vi "IniRW.vi"(6 "WriteIfNotExists":bool=TRUE, 7 "Operation":enum16{"None", "Read", "Write"}(ring)=enum."Read", 8 "InputValue":string, 9 "Key":string, 10 "Section":string, 11 "IniFilePath":path) -> (0 "IsValidFile":bool, 2 "OutputValue":string, 3 "IniFilePath out":path)   [LabVIEW 2024]
uses:
  <vilib>/Utility/config.llb/Read Key (String).vi
  <vilib>/Utility/config.llb/Write Key (String).vi
  <vilib>/Utility/config.llb/NI_LVConfig.lvlib
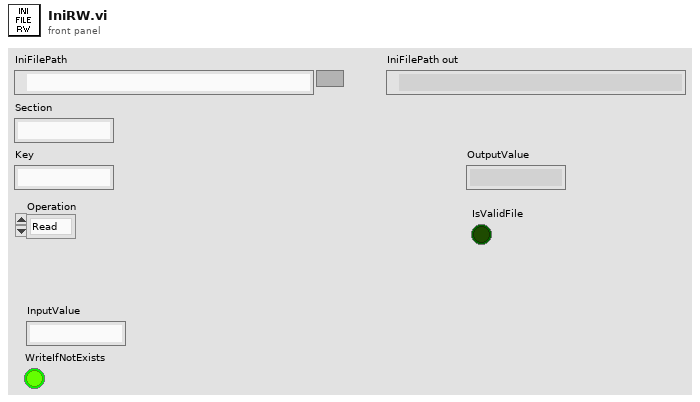
[diagram p1: front panel]
types:
  T1 = typedef "NI_LVConfig.lvlib/Config Data RefNum.ctl" = refnum<k1>
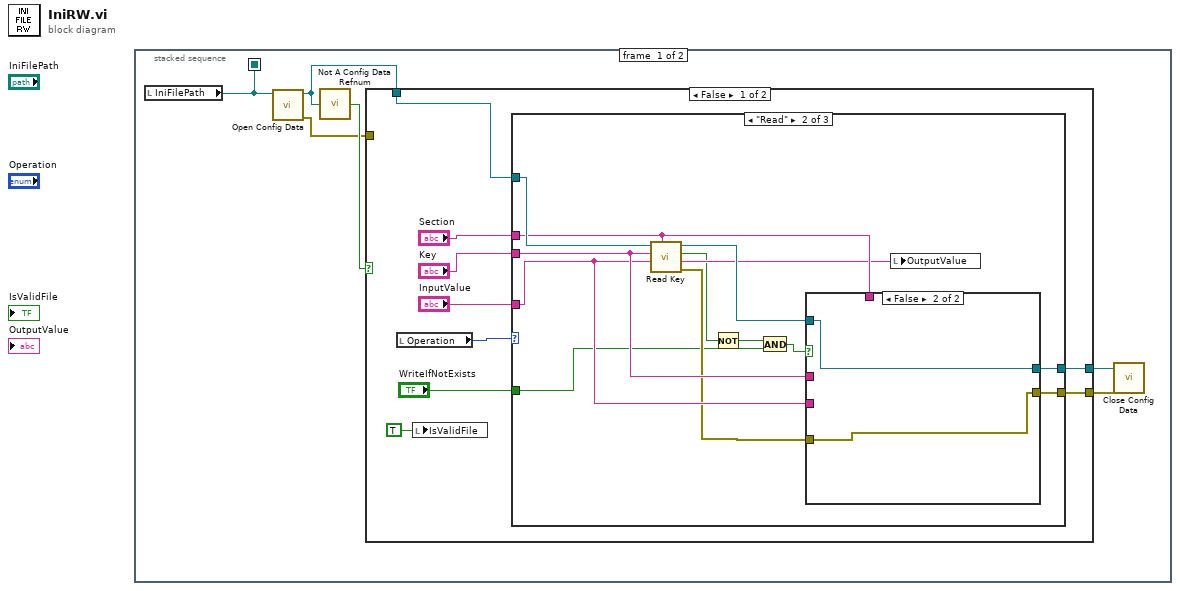
[diagram p0: block diagram]
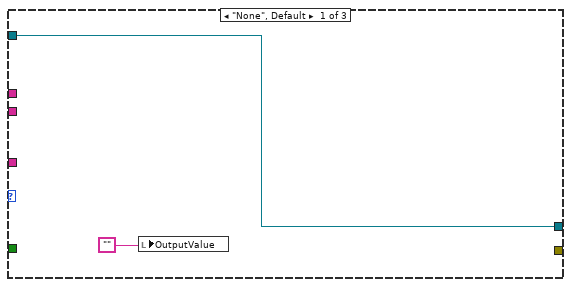
[diagram p2: hidden frame]
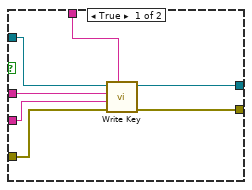
[diagram p3: hidden frame]
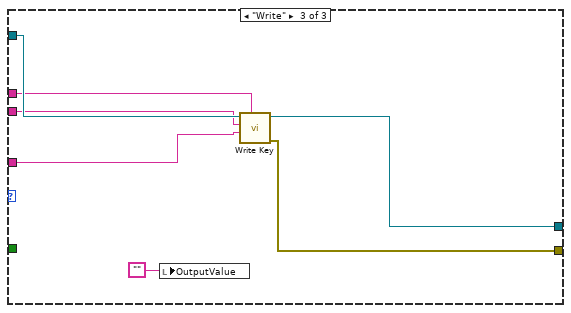
[diagram p4: hidden frame]
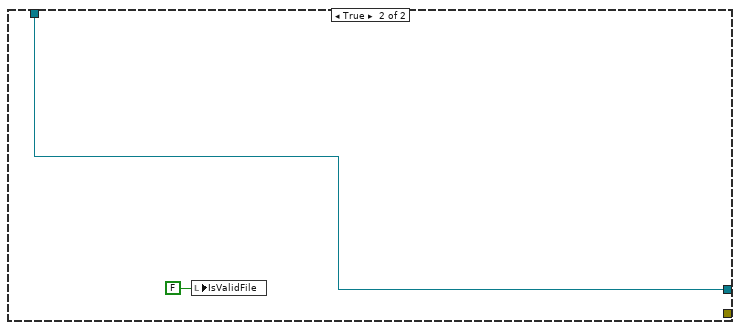
[diagram p5: hidden frame]
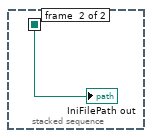
[diagram p6: hidden frame]
diagram:
  n1 = stacked-sequence {
    seq-local: [w1 _] -> [_ w49]
    frame #0 {
      n2 = local read "IniFilePath"() -> (w1:path)
      n3 = call <vilib>:"Open Config Data.vi"("configuration file path"=w1) -> ("error out"=w2:errorcluster, "refnum"=w5:T1)  [unwired: 8 in, 1 out]
      n4 = call <vilib>:"Not A Config Data Refnum.vi"("refnum"=w5) -> ("not a config data refnum"=w6:bool)
      n5 = case shown="False" w6 {
        tunnel: w5 -> [w13 w47]
        tunnel: [w9 w47] -> w4
        tunnel: [w8 _] -> w3
        tunnel: w2 -> [_ _]
        frame False {
          n6 = local read "Operation"() -> (w14:enum16{"None", "Read", "Write"})
          n7 = local write "IsValidFile"(TRUE ("IsValidFile")) -> ()
          n8 = case shown="\"Read\"" w14 {
            tunnel: w13 -> [w17 w30 w46]
            tunnel: "Section" -> [_ w28 w45]
            tunnel: "Key" -> [_ w27 w44]
            tunnel: "InputValue" -> [_ w26 w43]
            tunnel: [w17 w25 w41] -> w9
            tunnel: [_ w24 w42] -> w8
            tunnel: "WriteIfNotExists" -> [_ w19 _]
            frame "None", Default {
              n9 = local write "OutputValue"("") -> ()
            }
            frame "Read" {
              n10 = call-poly <vilib>:"Read Key.vi"("section"=w28, "default value"=w26, "key"=w27, "refnum"=w30) -> ("error out"=w22:errorcluster, "value"=w23:string, "found?"=w20:bool, "refnum out"=w29:T1)  [unwired: 4 in]
              n11 = Not(x=w20) -> (.not. x?=w18:bool)
              n12 = And(x=w18, y=w19) -> (x .and. y?=w21:bool)
              n13 = case shown="False" w21 {
                tunnel: w29 -> [w37 w39]
                tunnel: w28 -> [w36 _]
                tunnel: w27 -> [w35 _]
                tunnel: w26 -> [w34 _]
                tunnel: [w33 w39] -> w25
                tunnel: [w32 w38] -> w24
                tunnel: w22 -> [w31 w38]
                frame True {
                  n14 = call-poly <vilib>:"Write Key.vi"("section"=w36, "error in (no error)"=w31, "value"=w34, "key"=w35, "refnum"=w37) -> ("error out"=w32:errorcluster, "refnum out"=w33:T1)  [unwired: 4 in, 1 out]
                }
                frame False {
                }
              }
              n15 = local write "OutputValue"(w23) -> ()
            }
            frame "Write" {
              n16 = local write "OutputValue"("") -> ()
              n17 = call-poly <vilib>:"Write Key.vi"("section"=w45, "value"=w43, "key"=w44, "refnum"=w46) -> ("error out"=w42:errorcluster, "refnum out"=w41:T1)  [unwired: 5 in, 1 out]
            }
          }
        }
        frame True {
          n18 = local write "IsValidFile"(FALSE ("IsValidFile")) -> ()
        }
      }
      n19 = call <vilib>:"Close Config Data.vi"("error in (no error)"=w3, "refnum"=w4) -> ()  [unwired: 8 in, 2 out]
    }
    frame #1 {
      "IniFilePath out" <- w49
    }
  }
